vi "Validate Voltage.vi"(8 "error in (no error)":errorcluster, 10 "Voltage Setpoint in":dbl, 11 "Acopian in":refnum<class "Acopian.lvclass">) -> (0 "error out":errorcluster, 2 "Voltage Setpoint out":dbl, 3 "Acopian out":refnum<class "Acopian.lvclass">)   [LabVIEW 2019, in "Acopian.lvlib" / "Acopian.lvclass"]
uses:
  Library/Acopian.lvclass
  Library/Acopian.lvclass/Acopian.ctl
  Accessors/Read Max V.vi
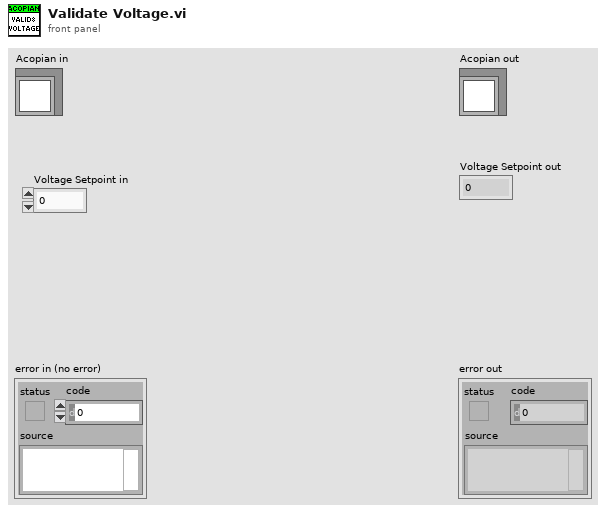
[diagram p1: front panel]
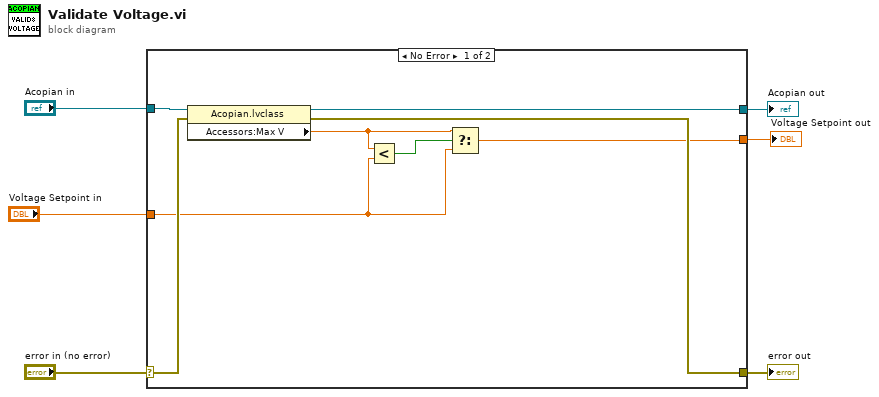
[diagram p0: block diagram]
diagram:
  n1 = case shown="No Error" "error in (no error)" {
    selector: "error in (no error)" -> [w12 w16]
    tunnel: [w9 w16] -> w5
    tunnel: [w10 w15] -> w3
    tunnel: "Acopian in" -> [w14 w15]
    tunnel: "Voltage Setpoint in" -> [w11 _]
    tunnel: [w8 _] -> w1
    frame No Error {
      n2 = property class="Acopian.lvclass"(reference=w14, error in=w12) -> (reference out=w10:refnum<class "Acopian.lvclass">, error out=w9:errorcluster, "Accessors:Max V"=w7:dbl)
      n3 = Less?(x=w7, y=w11) -> (x < y?=w13:bool)
      n4 = Select(t=w7, s=w13, f=w11) -> (s? t:f=w8:dbl)
    }
    frame Error {
    }
  }
  "error out" <- w5
  "Acopian out" <- w3
  "Voltage Setpoint out" <- w1
